vi "write2pipe.vi"() -> ()   [LabVIEW 2011]
panel:
  in  "text":string="kill"
  in  "path":path=path "/tmp/atlas/ambientpipe"
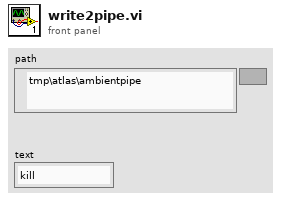
[diagram p1: front panel]
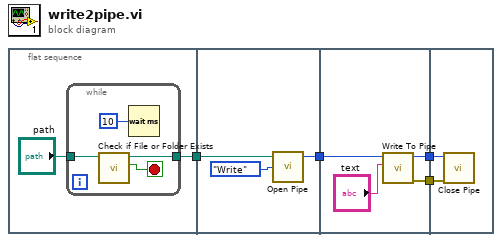
[diagram p0: block diagram]
diagram:
  n1 = flat-sequence {
    tunnel: [w5] -> w4
    tunnel: w4 -> [w13]
    tunnel: [w11] -> w3
    tunnel: w3 -> [w17]
    tunnel: [w15] -> w2
    tunnel: [w14] -> w1
    tunnel: w2 -> [w19]
    tunnel: w1 -> [w18]
    frame #0 {
      n2 = while {
        tunnel: "path" -> [w8]
        tunnel: [w7] -> w5
        stop <- w9 stop-if-true
        n3 = call <vilib>:"Check if File or Folder Exists.vi"("path"=w8) -> ("file or folder exists?"=w9:bool, "dup path"=w7:path)  [unwired: 8 in, 1 out]
        n4 = Wait (ms)(milliseconds to wait=u32 10) -> ()  [unwired: 1 out]
      }
    }
    frame #1 {
      n5 = call <vilib>:"Open Pipe.vi"("mode"=enum8{"Read", "Write"}."Write", "path to named pipe"=w13) -> ("file descriptor"=w11:i32)  [unwired: 2 in, 1 out]
    }
    frame #2 {
      n6 = call <vilib>:"Write To Pipe.vi"("data"="text", "file descriptor"=w17) -> ("error out"=w15:errorcluster, "file descriptor"=w14:i32)  [unwired: 3 in, 1 out]
    }
    frame #3 {
      n7 = call <vilib>:"Close Pipe.vi"("error in (no error)"=w19, "file descriptor"=w18) -> ()  [unwired: 4 in, 2 out]
    }
  }
